vi "Test_LSR_Transmission.vi"() -> ()   [LabVIEW 2015, in "LSR Transmission.lvlib"]
uses:
  LSR Transmission.lvlib
  Libraries/RDS Child Messages/MCB/MCB Motor Status.ctl
  Libraries/RDS Instruments/AIP/AIP Status.ctl
  Libraries/RDS Instruments/AIP/AIP States.ctl
  Actors/RDS Controller Actor/RDS Controller Actor/Controller.ctl
  Libraries/RDS Child Messages/Depth Data Message/Depth Data.ctl
  Libraries/RDS Instruments/Battery/Battery Data.ctl
  Libraries/RDS Child Messages/Battery Data/Battery Status.ctl
  Libraries/RDS Child Messages/Helm/Helm Status Message/Helm Status Control.ctl
  Actors/RDS Helm Actor/RDS Helm Actor/Helm State.ctl
  Libraries/RDS Child Messages/Helm/Heading Command/Heading Command Cntrl.ctl
  Libraries/RDS Child Messages/Helm/Steering Command/Steering Command Cntrl.ctl
  Libraries/RDS Child Messages/PID Gains/PID Gains Control.ctl
  Libraries/RDS Child Messages/Mission Messages/Mission Controller State Control.ctl
  RDS Mission Controller Actor/Mission Controller Navigation State.ctl
  RDS Mission Controller Actor/MissionOp.ctl
  Libraries/RDS Instruments/Compass/Compass Data.ctl
  Libraries/3rd Party/NMEA_GPS/NMEA_GPRMC-data.ctl
  Libraries/3rd Party/NMEA_GPS/NMEA_LatitudeDirection.ctl
  Libraries/3rd Party/NMEA_GPS/NMEA_LongitudeDirection.ctl
  Libraries/RDS Framework/RDS Message Class/RDS Message.lvclass
  RDS State Tracker/RDS State/RDS State.lvclass
  RDS State Tracker/RDS State/RDS State.lvclass/RDS State.ctl
  Libraries/RDS Framework/RDS Message Class/RDS Message.lvclass/RDS Message.ctl
  Libraries/RDS Child Messages/State Sample Message/State Sample Message.lvclass
  Libraries/RDS Child Messages/State Sample Message/State Sample Message.lvclass/State Sample Message.ctl
  RDS State Tracker/RDS State Tracker.lvlib
  Libraries/RDS Child Messages/RDS Child Messages.lvlib
  Libraries/RDS Instruments/RDS Instrument Library.lvlib
  Actors/RDS Controller Actor/RDS Controller Actor/RDS Controller Actor.lvlib
  Actors/RDS Helm Actor/RDS Helm Actor.lvlib
  RDS Mission Controller Actor/RDS Mission Controller Actor.lvlib
  Libraries/RDS Child Messages/Mission Messages/Mission Controller State Message.lvclass
  Libraries/3rd Party/NMEA_GPS/NMEA.lvlib
panel:
  out "Compressino Ratio":dbl[](graph)
  out "Time Unflatting":u32
  out "Time Unpacking":u32
  out "Time  Packing (ms)":u32
  out "Transmission":string
  out "Compression Ratio":dbl
  out "Compressed String":string
  out "Compressed Length":i32
  out "Transmission Complete?":bool
  out "data string":string
  out "Out":string
  out "Transmitted":i32
  out "Mission Controller State 2":T1 {"Mission"."GPS Longitude" format="%.6g"; "Mission"."GPS Latitude" format="%.6g"}
  out "Raw Length":i32
  in  "GPRMC-data":T4={"TimeStamp"=timestamp(0 s since 1904-01-01), "Validity"=FALSE, "Latitude"=0.0, "Latitude-Direction"=enum."North", "Longitude"=0.0, "Longitude-Direction"=enum."East", "Speed in knots"=0.0, "True course"=0.0, "Date Stamp"=timestamp(0 s since 1904-01-01), "Magnetic Variation (East/West)"=0.0, "GPS Latitude"=0.0, "GPS Longitude"=0.0} {"GPS Longitude" format="%.6f"; "GPS Latitude" format="%.6f"; "Magnetic Variation (East/West)" format="%.02f [deg]"; "Date Stamp" format="%<%x>T"; "True course" format="%.02f [deg]"; "Speed in knots" format="%.02f [kts]"; "Longitude" format="%0.4f [long]"; "Latitude" format="%.04f [lat]"; "TimeStamp" format="%<%.2X>T"}
  in  "Compass Data":T7
  in  "Port Motor Status":T8
  in  "Mission Controller State":T1 {"Mission"."GPS Longitude" format="%.6g"; "Mission"."GPS Latitude" format="%.6g"}
  in  "Helm Status":T9 {"Gains"."D (Td)" format="%#_9f"; "Gains"."I (Ti)" format="%#_9f"; "Gains"."P (Kc)" format="%#.9f"}
  in  "Battery Pack Info":T14
  in  "Depth Data":T16
  in  "Controller State":T17
  in  "AIP Status":T18
  in  "STBD Motor":T8
  # "Boat Side RDS State Creation"
  # "Transmission Process"
  # "Transmitted and Decoded RDS State"
  # "Unfortunately the LSR transmission is complicated for a couple of reasons:\n1.\tI need a transmission delimeter which means I need to use a byte stuffing technique called COBS\n2.\tCOBS has a max packet length of 254 so I need to split up a transmission into smaller packets\n3.\tA fully packet RDS transmission is pretty big and can be kilobytes long, so I implemented a compression technique that uses OpenG Zip tools."
  # "This part is empty cause i was too lazy to make the other ones. \nAlso not neceassary."
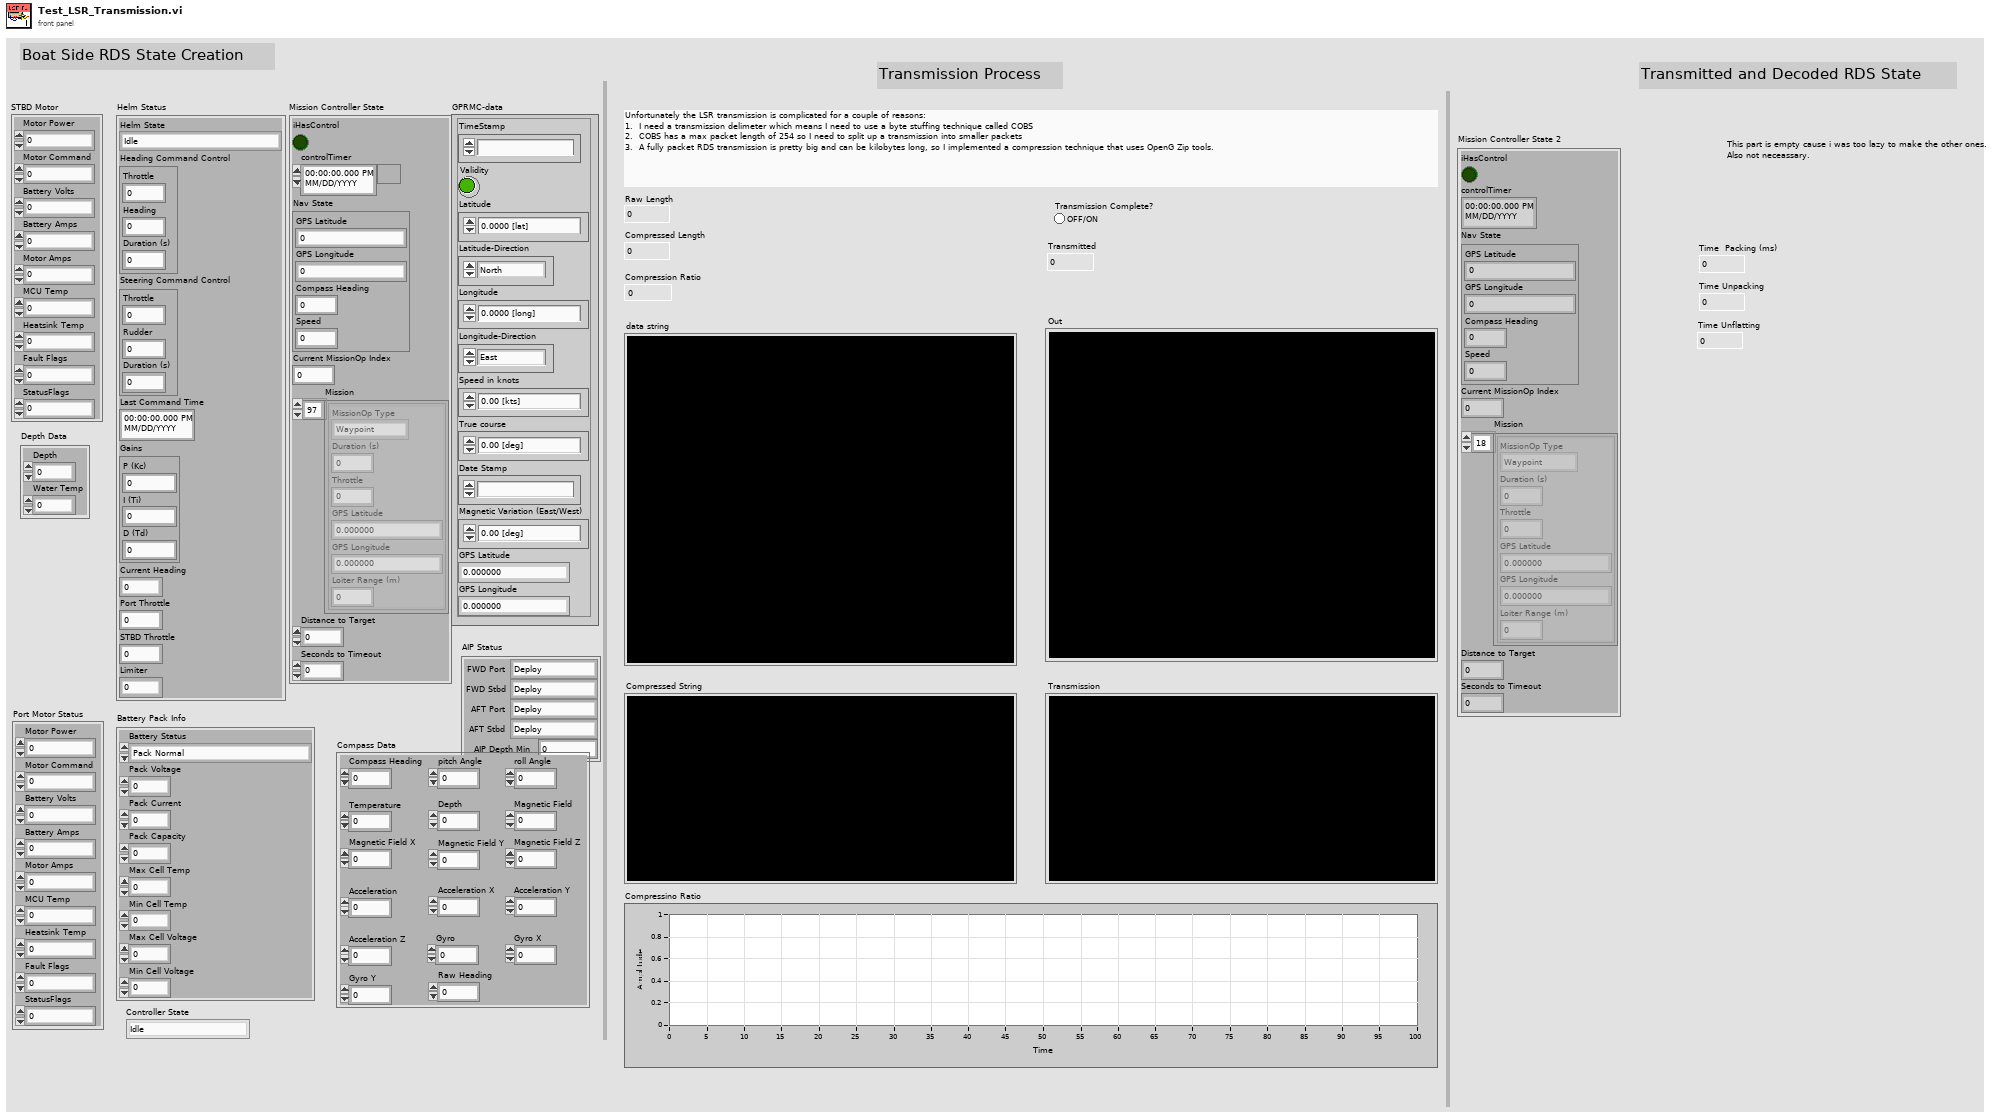
[diagram p1: front panel]
types:
  T1 = typedef "RDS Child Messages.lvlib/Mission Controller State Message.lvclass/Mission Controller State Control.ctl" = cluster{"iHasControl":bool, "controlTimer":timestamp, "Nav State":T2, "Current MissionOp Index":i32, "Mission":T3[], "Distance to Target":dbl, "Seconds to Timeout":dbl}
  T2 = typedef "RDS Mission Controller Actor.lvlib/Mission Controller Navigation State.ctl" = cluster{"GPS Latitude":ext, "GPS Longitude":ext, "Compass Heading":dbl, "Speed":dbl}
  T3 = typedef "RDS Mission Controller Actor.lvlib/MissionOp.ctl" = cluster{"MissionOp Type":enum16{"Waypoint", "Loiter", "Wait", "Deploy AIP", "Stow AIP"}, "Duration (s)":u16, "Throttle":i16, "GPS Latitude":dbl, "GPS Longitude":dbl, "Loiter Range (m)":u16}
  T4 = typedef "RDS Libraries.lvlib/NMEA.lvlib/NMEA_GPRMC-data.ctl" = cluster{"TimeStamp":timestamp, "Validity":bool, "Latitude":dbl, "Latitude-Direction":T5, "Longitude":dbl, "Longitude-Direction":T6, "Speed in knots":sgl, "True course":sgl, "Date Stamp":timestamp, "Magnetic Variation (East/West)":sgl, "GPS Latitude":dbl, "GPS Longitude":dbl}
  T5 = typedef "RDS Libraries.lvlib/NMEA.lvlib/NMEA_LatitudeDirection.ctl" = enum16{"", "North", "South"}
  T6 = typedef "RDS Libraries.lvlib/NMEA.lvlib/NMEA_LongitudeDirection.ctl" = enum16{"", "East", "West"}
  T7 = typedef "RDS Instrument Library.lvlib/Compass Data.ctl" = cluster{"Compass Heading":sgl, "pitch Angle":sgl, "roll Angle":sgl, "Temperature":sgl, "Depth":sgl, "Magnetic Field":sgl, "Magnetic Field X":sgl, "Magnetic Field Y":sgl, "Magnetic Field Z":sgl, "Acceleration":sgl, "Acceleration X":sgl, "Acceleration Y":sgl, "Gyro":sgl, "Gyro X":sgl, "Acceleration Z":sgl, "Gyro Y":sgl, "Raw Heading":sgl}
  T8 = typedef "RDS Child Messages.lvlib/MCB Motor Status.ctl" = cluster{"Motor Power":i16, "Motor Command":i16, "Battery Volts":sgl, "Battery Amps":sgl, "Motor Amps":sgl, "MCU Temp":i16, "Heatsink Temp":i16, "Fault Flags":u16, "StatusFlags":u16}
  T9 = typedef "RDS Child Messages.lvlib/Helm Status Control.ctl" = cluster{"Helm State":T10, "Heading Command Control":T11, "Steering Command Control":T12, "Last Command Time":timestamp, "Gains":T13, "Current Heading":dbl, "Port Throttle":i16, "STBD Throttle":i16, "Limiter":dbl}
  T10 = typedef "RDS Helm Actor.lvlib/Helm State.ctl" = enum16{"Idle", "Executing Heading Command", "Executing Steering Command"}
  T11 = typedef "RDS Child Messages.lvlib/Heading Command Cntrl.ctl" = cluster{"Throttle":i16, "Heading":sgl, "Duration (s)":i16}
  T12 = typedef "RDS Child Messages.lvlib/Steering Command Cntrl.ctl" = cluster{"Throttle":i16, "Rudder":i8, "Duration (s)":u16}
  T13 = typedef "RDS Child Messages.lvlib/PID Gains Control.ctl" = cluster{"P (Kc)":sgl, "I (Ti)":sgl, "D (Td)":sgl}
  T14 = typedef "RDS Instrument Library.lvlib/Battery Data.ctl" = cluster{"Battery Status":T15, "Pack Voltage":sgl, "Pack Current":sgl, "Pack Capacity":sgl, "Max Cell Temp":sgl, "Min Cell Temp":sgl, "Max Cell Voltage":sgl, "Min Cell Voltage":sgl}
  T15 = typedef "RDS Instrument Library.lvlib/Battery Status.ctl" = enum16{"Pack Normal", "Alarm: Cell temp too high", "Alarm: Pack voltage too high", "Warn: Pack voltage too high ", "Alarm: Pack voltage too low", "Warn: Pack voltage low", "Alarm Pack current too high", "Warn: Pack current too high ", "Fault: Pack to chassis connection detected", "Fault: Pack to cell connection error", "Fautl: System error"}
  T16 = typedef "RDS Child Messages.lvlib/Depth Data.ctl" = cluster{"Depth":sgl, "Water Temp":i8}
  T17 = typedef "RDS Controller Actor.lvlib/Controller.ctl" = enum16{"Idle", "Local Remote Control", "Shore Remote Control", "Mission Control"}
  T18 = typedef "RDS Instrument Library.lvlib/AIP Status.ctl" = cluster{"FWD Port":T19, "FWD Stbd":T19, "AFT Port":T19, "AFT Stbd":T19, "AIP Depth Min":u8}
  T19 = typedef "RDS Instrument Library.lvlib/AIP States.ctl" = enum16{"Deploy", "Deploying", "Deployed", "Stow", "Stowing", "Stowed", "Fault", "brakeOnStow", "breakOnDeploy", "Stopped", "Stopping"}
  T20 = typedef "RDS Child Messages.lvlib/RDS Message ID.ctl" = enum16{"RDS Hello World", "String Message", "AIP_Status", "AIP_Command", "GPS_Data", "MCB_Command", "MCB_Status", "Compass_Data", "Depth_Data", "Battery_Data", "Contoller_State", "Set_Mag_Dev", "BTB_Shutdown", "State_Sample_Request", "State_Sample", "PID_Gains_Set", "Helm_Limiter_Set", "Helm_Heading_Command", "Helm_Steering_Command", "Helm_Status", "Controller_Message", "AIP_Set_Min_Depth", "Mission_Controller_State", "Mission_Upload", "Mission_Set_Op_and_Run", "Mission_Settings_Set"}
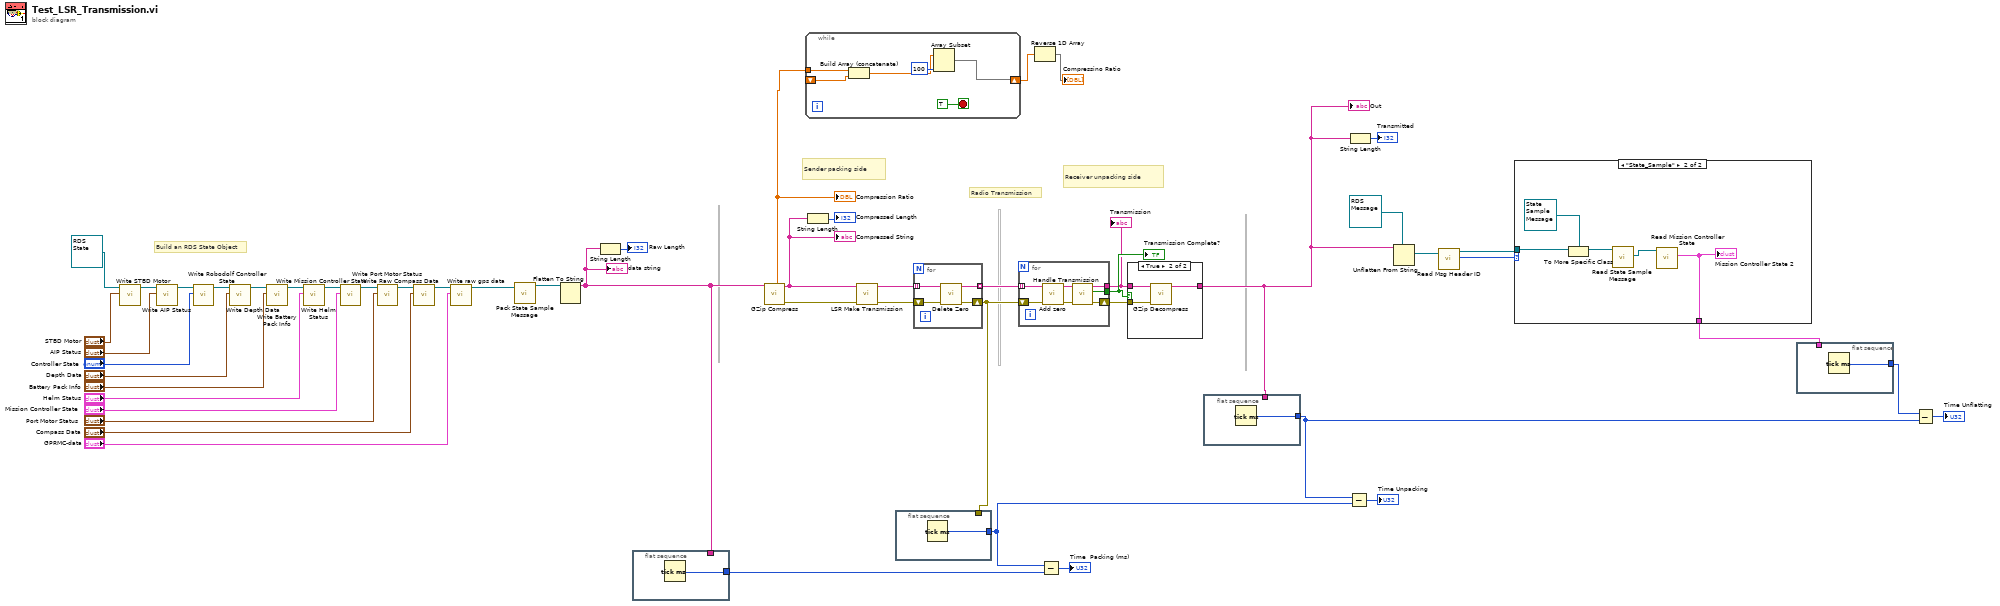
[diagram p0: block diagram]
diagram:
  # "Receiver unpacking side"
  # "Sender packing side"
  # "Radio Transmission"
  # "Build an RDS State Object"
  n1 = call "Write STBD Motor.vi"("STBD Motor"="STBD Motor", "RDS State in"=refnum<class "RDS State.lvclass"> refnum ("RDS State")) -> ("RDS State out"=w50:refnum<class "RDS State.lvclass">)  [unwired: 8 in, 1 out]
  n2 = call "Write AIP Status.vi"("AIP Status"="AIP Status", "RDS State in"=w50) -> ("RDS State out"=w49:refnum<class "RDS State.lvclass">)  [unwired: 8 in, 1 out]
  n3 = call "Write Robodolf Controller State.vi"("Controller State"="Controller State", "RDS State in"=w49) -> ("RDS State out"=w48:refnum<class "RDS State.lvclass">)  [unwired: 8 in, 1 out]
  n4 = call "Write Depth Data.vi"("Depth Data"="Depth Data", "RDS State in"=w48) -> ("RDS State out"=w47:refnum<class "RDS State.lvclass">)  [unwired: 8 in, 1 out]
  n5 = call "Write Battery Pack Info.vi"("Battery Pack Info"="Battery Pack Info", "RDS State in"=w47) -> ("RDS State out"=w46:refnum<class "RDS State.lvclass">)  [unwired: 8 in, 1 out]
  n6 = call "Write Helm Status.vi"("Helm Status"="Helm Status", "RDS State in"=w46) -> ("RDS State out"=w45:refnum<class "RDS State.lvclass">)  [unwired: 8 in, 1 out]
  n7 = call "Write Mission Controller State.vi"("Mission Controller State"="Mission Controller State", "RDS State in"=w45) -> ("RDS State out"=w44:refnum<class "RDS State.lvclass">)  [unwired: 8 in, 1 out]
  n8 = call "Write Port Motor Status.vi"("Port Motor Status"="Port Motor Status", "RDS State in"=w44) -> ("RDS State out"=w43:refnum<class "RDS State.lvclass">)  [unwired: 8 in, 1 out]
  n9 = call "Write Raw Compass Data.vi"("Compass Data"="Compass Data", "RDS State in"=w43) -> ("RDS State out"=w42:refnum<class "RDS State.lvclass">)  [unwired: 8 in, 1 out]
  n10 = call "Write raw gps data.vi"("GPRMC-data"="GPRMC-data", "RDS State in"=w42) -> ("RDS State out"=w27:refnum<class "RDS State.lvclass">)  [unwired: 8 in, 1 out]
  n11 = call "Pack State Sample Message.vi"("State Sample"=w27) -> ("State Sample Message out"=w26:refnum<class "State Sample Message.lvclass">)  [unwired: 10 in]
  n12 = Flatten To String(anything=w26) -> (data string=w14:string)  [unwired: 3 in, 2 out]
  "data string" <- w14
  n13 = String Length(string=w14) -> (length=→"Raw Length":i32)
  n14 = flat-sequence {
    tunnel: w14 -> [_]
    tunnel: [w52] -> w10
    frame #0 {
      n15 = Tick Count (ms)() -> (millisecond timer value=w52:u32)
    }
  }
  n16 = call "GZip Compress.vi"("Uncompressed string"=w14) -> ("error out"=w21:errorcluster, "GZip compressed string"=w17:string, "Ratio"=w3:dbl)  [unwired: 8 in]
  "Compressed String" <- w17
  "Compression Ratio" <- w3
  n17 = while {
    shift-right: [w54] -> w2
    shift-left: _ -> [w57]
    tunnel: w3 -> [w53]
    stop <- TRUE stop-if-true
    n18 = Build Array (concatenate)(w53, w57) -> (w55:dbl[])
    n19 = Array Subset(array=w55, length=100) -> (w54:dbl[])  [unwired: 1 in]
  }
  n20 = String Length(string=w17) -> (length=→"Compressed Length":i32)
  n21 = call "LSR Make Transmission.vi"("error in (no error)"=w21, "Data String"=w17) -> ("error out"=w24:errorcluster, "Transmission"=w25:string[])  [unwired: 8 in]
  n22 = flat-sequence {
    tunnel: [w59] -> w8
    tunnel: w13 -> [_]
    frame #0 {
      n23 = Tick Count (ms)() -> (millisecond timer value=w59:u32)
    }
  }
  n24 = for {
    tunnel: w25 -> [w63] mode=indexing
    tunnel: [w61] -> w22 mode=indexing
    shift-right: [w60] -> w13
    shift-left: w24 -> [w62]
    n25 = call "Delete Zero.vi"("error in (no error)"=w62, "COBS String in"=w63) -> ("error out"=w60:errorcluster, "String out"=w61:string)  [unwired: 8 in]
  }
  n26 = for {
    tunnel: [w69] -> w16
    tunnel: [w68] -> w15
    tunnel: w22 -> [w67] mode=indexing
    shift-right: [w70] -> w20
    shift-left: w13 -> [w64]
    n27 = call "Add zero.vi"("error in (no error)"=w64, "String in"=w67) -> ("error out"=w65:errorcluster, "String out"=w66:string)  [unwired: 8 in]
    n28 = call "Handle Transmission.vi"("error in (no error)"=w65, "Stuffed Data"=w66) -> ("error out"=w70:errorcluster, "Transmission valid?"=w69:bool, "Transmission"=w68:string)  [unwired: 7 in]
  }
  "Transmission Complete?" <- w16
  "Transmission" <- w15
  n29 = Reverse 1D Array(array=w2) -> (reversed array=→"Compressino Ratio":dbl[])
  n30 = Subtract(x=w8, y=w10) -> (x-y=→"Time  Packing (ms)":u32)
  n31 = case shown="True" w16 {
    tunnel: [w71 w74] -> w12
    tunnel: w15 -> [w71 w73]
    tunnel: w20 -> [_ w72]
    frame False {
    }
    frame True {
      n32 = call "GZip Decompress.vi"("error in (no error)"=w72, "GZip compressed string"=w73) -> ("Decompressed string"=w74:string)  [unwired: 8 in, 1 out]
    }
  }
  "Out" <- w12
  n33 = flat-sequence {
    tunnel: [w75] -> w4
    tunnel: w12 -> [_]
    frame #0 {
      n34 = Tick Count (ms)() -> (millisecond timer value=w75:u32)
    }
  }
  n35 = Subtract(x=w4, y=w8) -> (x-y=→"Time Unpacking":u32)
  n36 = String Length(string=w12) -> (length=→"Transmitted":i32)
  n37 = Unflatten From String(type=refnum<class "RDS Message.lvclass"> refnum ("RDS Child Messages.lvlib:RDS Message.lvclass"), binary string=w12) -> (value=w29:refnum<class "RDS Message.lvclass">)  [unwired: 3 in, 2 out]
  n38 = call "Read Msg Header ID.vi"("RDS Message in"=w29) -> ("Msg ID"=w28:T20, "RDS Message out"=w19:refnum<class "RDS Message.lvclass">)  [unwired: 6 in, 3 out]
  n39 = case shown="\"State_Sample\"" w28 {
    tunnel: w19 -> [_ w79]
    tunnel: [_ w76] -> w11
    frame "RDS Hello World", Default {
    }
    frame "State_Sample" {
      n40 = To More Specific Class(target class=refnum<class "State Sample Message.lvclass"> refnum ("State Sample Message out"), reference=w79) -> (specific class reference=w77:refnum<class "State Sample Message.lvclass">)  [unwired: 1 in, 1 out]
      n41 = call "Read State Sample Message.vi"("State Sample Message in"=w77) -> ("State Sample"=w80:refnum<class "RDS State.lvclass">)  [unwired: 8 in, 2 out]
      n42 = call "Read Mission Controller State.vi"("RDS State in"=w80) -> ("Mission Controller State"=w76:T1)  [unwired: 8 in, 2 out]
      "Mission Controller State 2" <- w76
    }
  }
  n43 = flat-sequence {
    tunnel: [w81] -> w5
    tunnel: w11 -> [_]
    frame #0 {
      n44 = Tick Count (ms)() -> (millisecond timer value=w81:u32)
    }
  }
  n45 = Subtract(x=w5, y=w4) -> (x-y=→"Time Unflatting":u32)
